vi "GetParam.vi"(8 "error in (no error)":errorcluster caption="entrée d'erreur (pas d'erreur)", 11 "Binarizer en entrée":refnum<class "Binarizer.lvclass">) -> (0 "error out":errorcluster caption="sortie d'erreur", 2 "Binarizer":cluster{"threshold":dbl, "copy":bool}={"threshold"=0.0, "copy"=TRUE}, 3 "Binarizer en sortie":refnum<class "Binarizer.lvclass">)   [LabVIEW 2020, in "Binarizer.lvclass"]
doc: "Get Parameters"
uses:
  Binarizer.lvclass
  Binarizer.lvclass/Binarizer.ctl
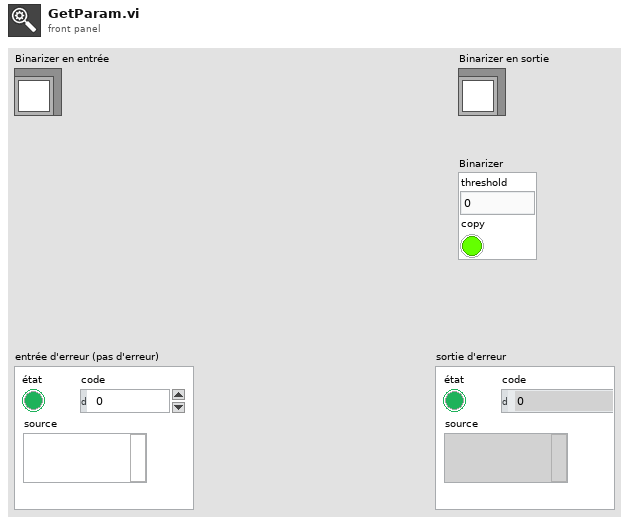
[diagram p1: front panel]
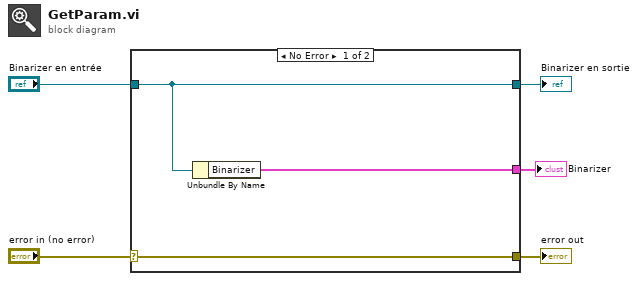
[diagram p0: block diagram]
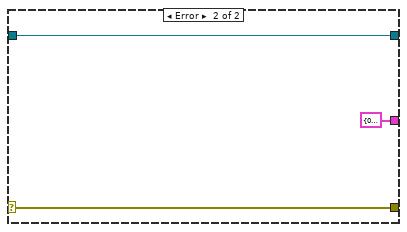
[diagram p2: hidden frame]
diagram:
  n1 = case shown="No Error" "error in (no error)" {
    selector: "error in (no error)" -> [w8 w10]
    tunnel: [w8 w10] -> w4
    tunnel: [w7 w11] -> w2
    tunnel: "Binarizer en entrée" -> [w7 w11]
    tunnel: [w6 cluster{"threshold":dbl, "copy":bool} {"threshold"=0.0, "copy"=FALSE} ("Binarizer")] -> w1
    frame No Error {
      n2 = Unbundle By Name(w7) -> ("Binarizer"=w6:cluster{"threshold":dbl, "copy":bool})
    }
    frame Error {
    }
  }
  "error out" <- w4
  "Binarizer en sortie" <- w2
  "Binarizer" <- w1
